vi "NISE.local.Read Register (Core).vi"(0 "SLSC Local in":refnum<class "SLSC Interface.lvclass">, 1 "type":enum16{"U8", "U16", "U32", "U64"}(ring), 5 "device":refnum<k21>="$DefaultDevices", 7 "register address":u32 format="%.0x", 11 "error in (no error)":errorcluster) -> (4 "SLSC Local out":refnum<class "SLSC Interface.lvclass">, 6 "device out":refnum<k21>, 8 "next register address":u32 format="%.0x", 10 "data out":u64 format="%.0x", 15 "error out":errorcluster)   [LabVIEW 2016, in "SLSC Interface.lvclass"]
uses:
  SLSC Interface Class/SLSC Interface.lvclass
  SLSC Interface Class/NISE.Read session.vi
  <vilib>/SLSC/Read Register (U64).vi
  <vilib>/SLSC/Read Register (U32).vi
  <vilib>/SLSC/Read Register (U16).vi
  <vilib>/SLSC/Read Register (U8).vi
  SLSC Interface Class/NISE.Write session.vi
  <vilib>/SLSC/SLSC.lvlib
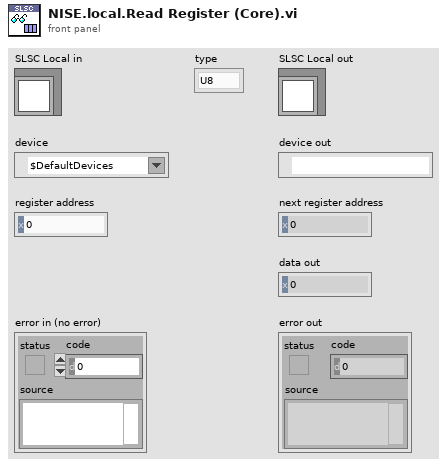
[diagram p1: front panel]
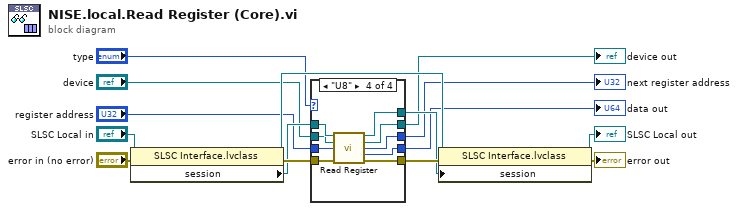
[diagram p0: block diagram]
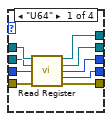
[diagram p2: hidden frame]
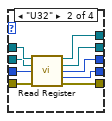
[diagram p3: hidden frame]
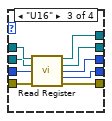
[diagram p4: hidden frame]
diagram:
  n1 = property class="SLSC Interface.lvclass"(reference="SLSC Local in", error in="error in (no error)") -> (reference out=w13:refnum<class "SLSC Interface.lvclass">, error out=w15:errorcluster, "session"=w12:refnum<k21>)
  n2 = case shown="\"U8\"" "type" {
    tunnel: w15 -> [w24 w33 w42 w51]
    tunnel: [w23 w32 w41 w50] -> w14
    tunnel: w12 -> [w22 w31 w40 w49]
    tunnel: [w21 w30 w39 w48] -> w11
    tunnel: "device" -> [w20 w29 w38 w47]
    tunnel: "register address" -> [w19 w28 w37 w46]
    tunnel: [w18 w27 w36 w45] -> w6
    tunnel: [w17 w26 w35 w44] -> w5
    tunnel: [w16 w25 w34 w43] -> w4
    frame "U64" {
      n3 = call-poly <vilib>:"Read Register.vi"("session in"=w22, "device"=w20, "register address"=w19, "error in (no error)"=w24) -> ("session out"=w21:refnum<k21>, "device out"=w16:refnum<k21>, "next register address"=w17:u32, "data out"=w18:u64, "error out"=w23:errorcluster)  [unwired: 7 in]
    }
    frame "U32" {
      n4 = call-poly <vilib>:"Read Register.vi"("session in"=w31, "device"=w29, "register address"=w28, "error in (no error)"=w33) -> ("session out"=w30:refnum<k21>, "device out"=w25:refnum<k21>, "next register address"=w26:u32, "data out"=w27:u32, "error out"=w32:errorcluster)  [unwired: 7 in]
    }
    frame "U16" {
      n5 = call-poly <vilib>:"Read Register.vi"("session in"=w40, "device"=w38, "register address"=w37, "error in (no error)"=w42) -> ("session out"=w39:refnum<k21>, "device out"=w34:refnum<k21>, "next register address"=w35:u32, "data out"=w36:u16, "error out"=w41:errorcluster)  [unwired: 7 in]
    }
    frame "U8" {
      n6 = call-poly <vilib>:"Read Register.vi"("session in"=w49, "device"=w47, "register address"=w46, "error in (no error)"=w51) -> ("session out"=w48:refnum<k21>, "device out"=w43:refnum<k21>, "next register address"=w44:u32, "data out"=w45:u8, "error out"=w50:errorcluster)  [unwired: 7 in]
    }
  }
  "device out" <- w4
  "next register address" <- w5
  "data out" <- w6
  n7 = property class="SLSC Interface.lvclass"(reference=w13, error in=w14, "session"=w11) -> (reference out=→"SLSC Local out":refnum<class "SLSC Interface.lvclass">, error out=→"error out":errorcluster)
